vi "Dodaj_kursor_WFM.vi"(7 "Wektor przebiegow":waveform(dbl)[](array[waveform]), 8 "error in (no error)":errorcluster, 11 "Wykres Ref":refnum<vi>) -> (0 "error out":errorcluster)   [LabVIEW 2013]
doc: "Dodaje kursor do wskaŸnika wyktesu\nWavefogm Graph"
uses:
  <vilib>/measure/NI_MABase.lvlib
panel:
  in  "Array":T1(array[cluster])=[{"signal type"=enum."Sine Wave", "frequency"=10.0, "amplitude"=2.0}, {"signal type"=enum."Sine Wave", "frequency"=13.0, "amplitude"=1.0}, {"signal type"=enum."Sine Wave", "frequency"=7.0, "amplitude"=1.0}, {"signal type"=enum."Sine Wave", "frequency"=5.0, "amplitude"=3.0}] {"amplitude" format="%0.2p"; "frequency" format="%0.2p"}
  in  "Styl punktu":u8=11 max=16 step=1
  in  "Nazwa on":bool=TRUE
  in  "Styl kursora":u8=4 max=8 step=1
  in  "Cancel":bool
  in  "OK":bool
  in  "Kolor":u32(colorbox)=16776704
  in  "Nazwa":string="Kursor"
  in  "Typ Kursora":T2(tab)=enum."Jeden przebieg"
  in  "Monitorowany przebieg":i32(ring) items=["Przebieg 0", "Przebieg 1", "Przebieg 2", "Przebieg 3"]
  in  "Monitoruj wszystkie przebiegi":bool
  in  "Drugi monitorowany przebieg":i32(ring) items=["Przebieg 0", "Przebieg 1", "Przebieg 2", "Przebieg 3"]
  in  "Pierwszy monitorowany przebieg":i32(ring) items=["Przebieg 0", "Przebieg 1", "Przebieg 2", "Przebieg 3"]
  # "Style kursora:"
  # "Typy punktu kursora:"
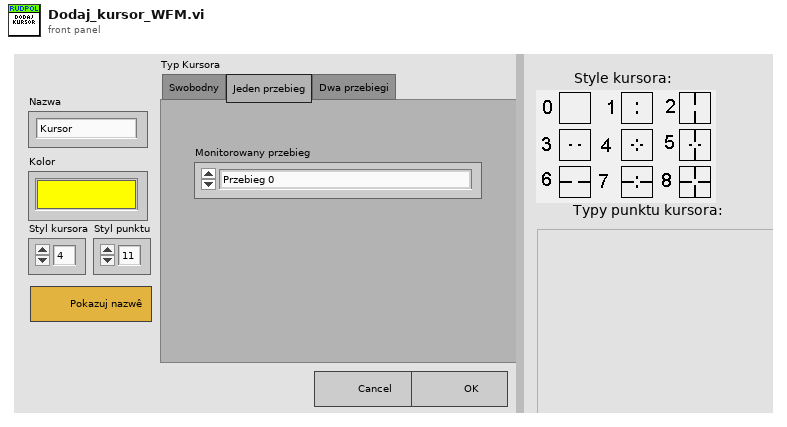
[diagram p1: front panel]
types:
  T1 = cluster{"signal type":enum16{"Sine Wave", "Triangle Wave", "Square Wave", "Sawtooth Wave"}, "frequency":dbl, "amplitude":dbl}[]
  T2 = enum32{"Swobodny", "Jeden przebieg", "Dwa przebiegi"}
  T3 = enum16{"Sine Wave", "Triangle Wave", "Square Wave", "Sawtooth Wave"}
  T4 = cluster{"Name":string, "Color":u32, "Style":u8, "Point Style":u8, "Name Visible":bool, "Allow Drag":bool, "Cursor Mode":u32, "Plot":i32, "Index":i32, "Position":cluster{"X":dbl, "Y":dbl}, "X Scale":u32, "Y Scale":u32, "Watch Plots":i32[], "Watch All Plots":bool, "Plot Area":i32, "Label Offset":cluster{"X":dbl, "Y":dbl}}
  T5 = typedef "LVCursorListTypeDef.ctl" = cluster{"Name":string, "Color":u32, "Style":u8, "Point Style":u8, "Name Visible":bool, "Allow Drag":bool, "Cursor Mode":u32, "Plot":i32, "Index":i32, "Position":cluster{"X":dbl, "Y":dbl}, "X Scale":u32, "Y Scale":u32, "Watch Plots":i32[], "Watch All Plots":bool, "Plot Area":i32, "Label Offset":cluster{"X":dbl, "Y":dbl}}[]
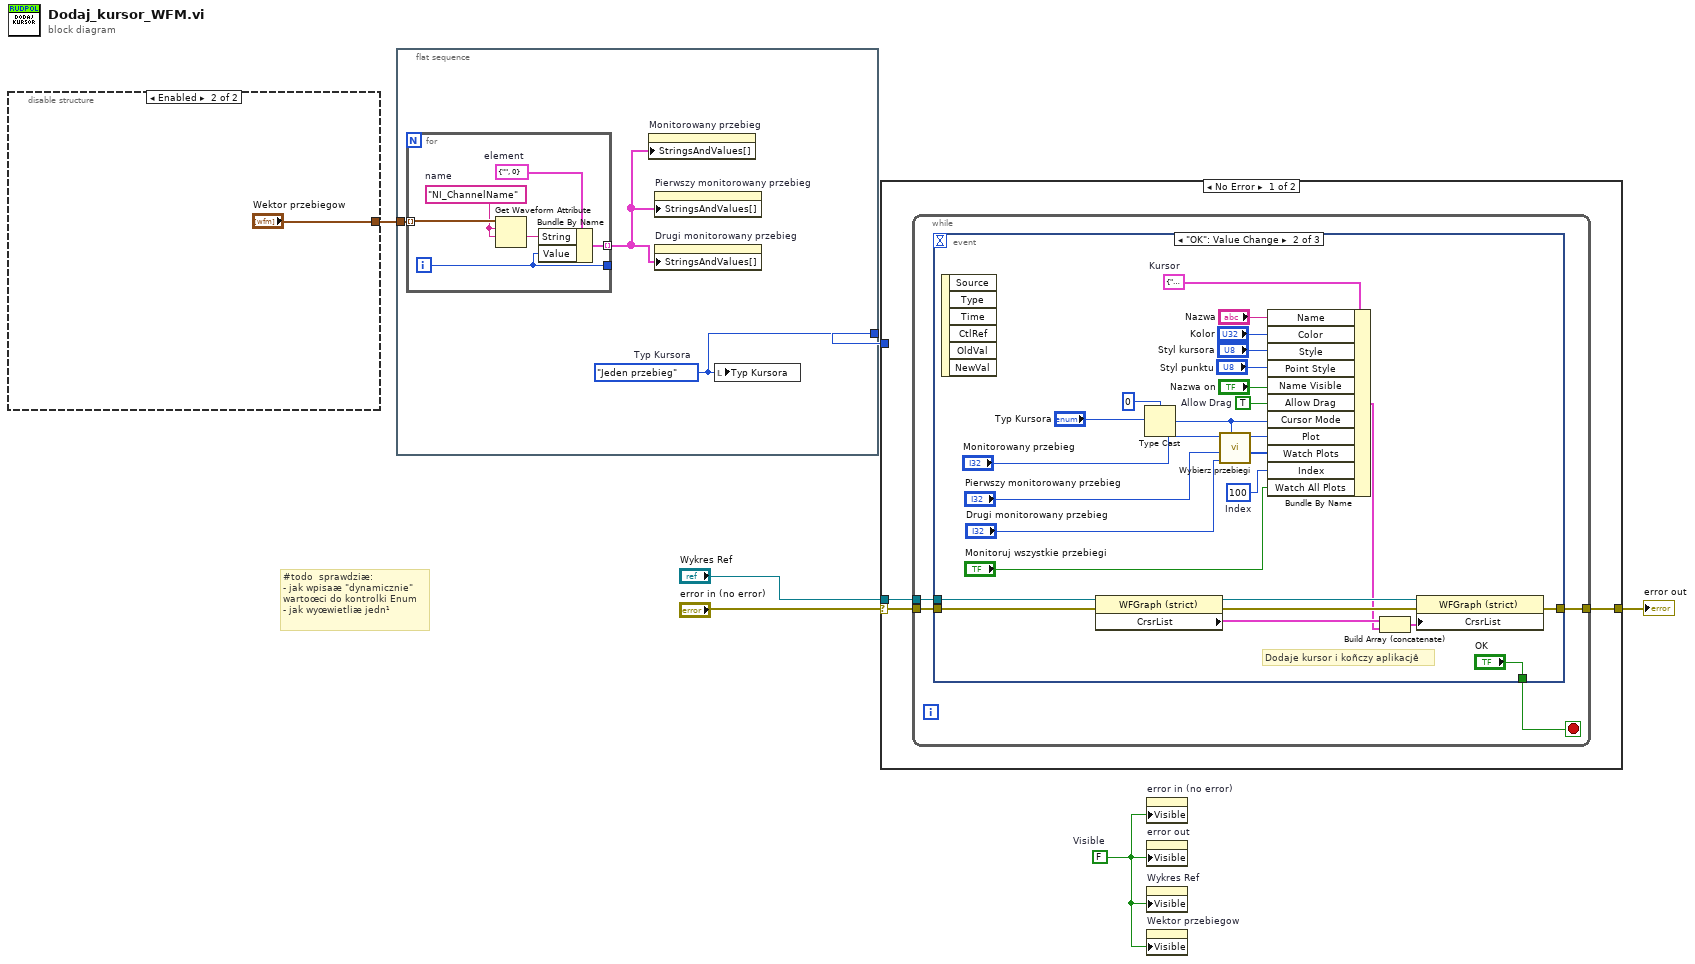
[diagram p0: block diagram]
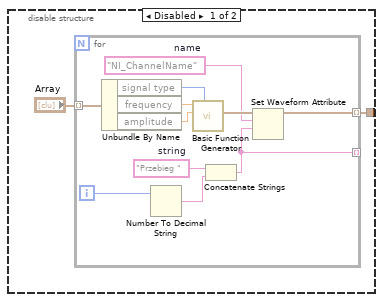
[diagram p2: hidden frame]
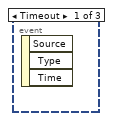
[diagram p3: hidden frame]
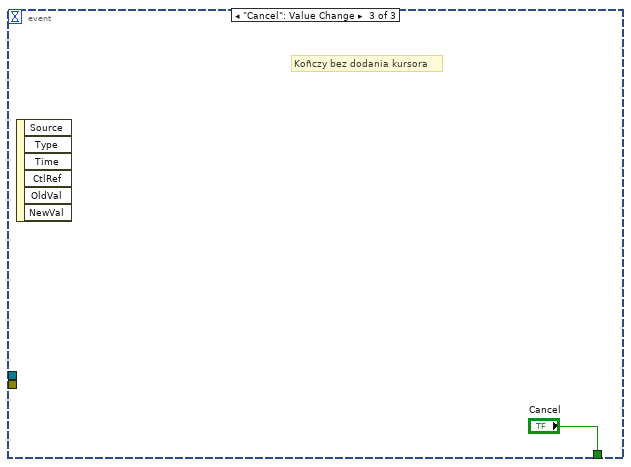
[diagram p4: hidden frame]
diagram:
  w3 = FALSE  # Visible
  # "#todo  sprawdziæ:\n- jak wpisaæ \"dynamicznie\"\nwartoœci do kontrolki Enum\n- jak wyœwietliæ jedn¹"
  n1 = disable-structure shown="Enabled" {
    disable-tunnel: [w7 "Wektor przebiegow"] -> w1
    frame Disabled {
      n2 = for {
        tunnel: "Array" -> [w16] mode=indexing
        tunnel: [w10] -> w7 mode=indexing
        tunnel: [w9] -> _ mode=indexing
        i -> [w11]
        w13 = "Przebieg "  # string
        w14 = "NI_ChannelName"  # name
        n3 = Unbundle By Name(w16) -> ("signal type"=w19:T3, "frequency"=w18:dbl, "amplitude"=w17:dbl)
        n4 = Number To Decimal String(number=w11) -> (decimal integer string=w12:string)  [unwired: 1 in]
        n5 = call <vilib>:"Basic Function Generator.vi"("signal type"=w19, "amplitude"=w17, "frequency"=w18) -> ("signal out"=w15:waveform(dbl))  [unwired: 6 in, 2 out]
        n6 = Concatenate Strings(w13, w12) -> (w9:string)
        n7 = Set Waveform Attribute(5:w9, 6:w14, 7:w15) -> (3:w10:waveform(dbl))  [unwired: 1 in, 2 out]
      }
    }
    frame Enabled {
    }
  }
  n8 = flat-sequence {
    tunnel: [w23] -> w2
    tunnel: w1 -> [w22]
    frame #0 {
      w23 = T2."Jeden przebieg"  # Typ Kursora
      n9 = for {
        tunnel: w22 -> [w29] mode=indexing
        tunnel: [w25] -> _
        tunnel: [w24] -> w21 mode=indexing
        i -> [w25]
        w27 = cluster{"String":string, "Value":u16} {"String"="", "Value"=0}  # element
        w28 = "NI_ChannelName"  # name
        n10 = Get Waveform Attribute(5:w28, 6:w28, 7:w29) -> (1:w26:string)  [unwired: 1 in, 3 out]
        n11 = Bundle By Name(cluster=w27, "String"=w26, "Value"=w25) -> (w24:cluster{"String":string, "Value":u16})
      }
      n12 = property on="Monitorowany przebieg" class="Ring (strict)"("StringsAndValues[]"=w21) -> ()  [unwired: 2 in, 2 out]
      n13 = property on="Pierwszy monitorowany przebieg" class="Ring (strict)"("StringsAndValues[]"=w21) -> ()  [unwired: 2 in, 2 out]
      n14 = property on="Drugi monitorowany przebieg" class="Ring (strict)"("StringsAndValues[]"=w21) -> ()  [unwired: 2 in, 2 out]
      n15 = local write "Typ Kursora"(w23) -> ()
    }
  }
  n16 = case shown="No Error" "error in (no error)" {
    selector: "error in (no error)" -> [w32 w64]
    tunnel: [w31 w64] -> w5
    tunnel: "Wykres Ref" -> [w30 _]
    tunnel: w2 -> [_ _]
    frame No Error {
      n17 = while {
        tunnel: w32 -> [w34]
        tunnel: [w33] -> w31
        tunnel: w30 -> [w36]
        stop <- w35 stop-if-true
        n18 = event shown="[1] \"OK\": Value Change" {
          selector: _ -> [_ _ _]
          dyn-events: _ -> [_ _ _]
          timeout: _ -> [_ _ _]
          tunnel: w36 -> [_ w61 _]
          tunnel: [_ "OK" "Cancel"] -> w35
          tunnel: w34 -> [_ w60 _]
          tunnel: [_ w57 _] -> w33
          event Timeout {
            n19 = event-data() -> ()  [unwired: 1 in, 3 out]
          }
          event "OK": Value Change {
            w38 = 100  # Index
            w47 = TRUE  # Allow Drag
            w54 = T4 {"Name"="", "Color"=0, "Style"=0, "Point Style"=0, "Name Visible"=FALSE, "Allow Drag"=FALSE, "Cursor Mode"=0, "Plot"=0, "Index"=0, "Position"={"X"=0.0, "Y"=0.0}, "X Scale"=0, "Y Scale"=0, "Watch Plots"=[], "Watch All Plots"=FALSE, "Plot Area"=0, "Label Offset"={"X"=0.0, "Y"=0.0}}  # Kursor
            # "Dodaje kursor i koñczy aplikacjê"
            n20 = event-data() -> ()  [unwired: 1 in, 6 out]
            n21 = property class="WFGraph (strict)"(reference=w61, error in=w60) -> (reference out=w59:refnum<vi>, error out=w58:errorcluster, "CrsrList"=w56:T5)
            n22 = Type Cast(type=u32 0, x="Typ Kursora") -> (*(type *) &x=w42:u32)
            n23 = call "Wybierz przebiegi.vi"("Mode"=w42, "Wybierz drugi monitorowanyprzebieg"="Drugi monitorowany przebieg", "Wybierz pierwszy monitorowanyprzebieg"="Pierwszy monitorowany przebieg", "Wybierz monitorowany przebieg"="Monitorowany przebieg") -> ("WPlots"=w43:i32[], "Plot"=w44:i32)  [unwired: 6 in]
            n24 = Bundle By Name(cluster=w54, "Name"="Nazwa", "Color"="Kolor", "Style"="Styl kursora", "Point Style"="Styl punktu", "Name Visible"="Nazwa on", "Allow Drag"=w47, "Cursor Mode"=w42, "Plot"=w44, "Watch Plots"=w43, "Index"=w38, "Watch All Plots"="Monitoruj wszystkie przebiegi") -> (w53:T4)
            n25 = Build Array (concatenate)(w56, w53) -> (w55:T5)
            n26 = property class="WFGraph (strict)"(reference=w59, error in=w58, "CrsrList"=w55) -> (error out=w57:errorcluster)  [unwired: 1 out]
          }
          event "Cancel": Value Change {
            # "Koñczy bez dodania kursora"
            n27 = event-data() -> ()  [unwired: 1 in, 6 out]
          }
        }
      }
    }
    frame Error {
    }
  }
  "error out" <- w5
  n28 = property on="error in (no error)" class="Clust (strict)"("Visible"=w3) -> ()  [unwired: 2 in, 2 out]
  n29 = property on="error out" class="Clust (strict)"("Visible"=w3) -> ()  [unwired: 2 in, 2 out]
  n30 = property on="Wykres Ref" class="LVObjRef (strict)"("Visible"=w3) -> ()  [unwired: 2 in, 2 out]
  n31 = property on="Wektor przebiegow" class="Arr (strict)"("Visible"=w3) -> ()  [unwired: 2 in, 2 out]
